vi "Open_abscisseSD.vi"(1 "wavelengths path":path) -> (0 "wavelengths":dbl[](array[numeric]) format="%.4f")   [LabVIEW 2015]
uses:
  <vilib>/Utility/file.llb/Read Delimited Spreadsheet (DBL).vi
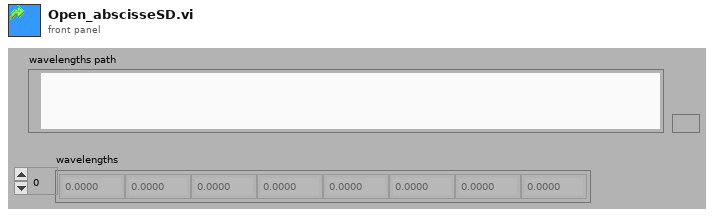
[diagram p1: front panel]
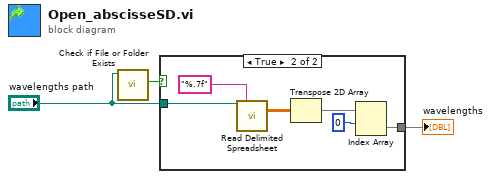
[diagram p0: block diagram]
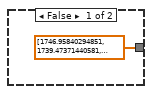
[diagram p2: hidden frame]
diagram:
  n1 = call <vilib>:"Check if File or Folder Exists.vi"("path"="wavelengths path") -> ("file or folder exists?"=w2:bool)  [unwired: 8 in, 2 out]
  n2 = case shown="True" w2 {
    tunnel: "wavelengths path" -> [_ w10]
    tunnel: [dbl[] [1746.95840294851, 1739.47371440581, 1731.99263543554, 1724.5156950524101, 1717.04336159476, 1709.5761853721801, 1702.1146510360302, 1694.65931938089, 1687.21070135242, 1679.76935602013, 1672.33583286395, 1664.91067290181, 1657.4944812369401, 1650.08777499183, 1642.69118936313, 1635.30526816863, 1627.93059787024, 1620.5678256451802, 1613.2174869458, 1605.8802162495501, 1598.55664914169, 1591.2473459440598, 1583.95293766588, 1576.67410341541, 1569.41139768648, 1562.16544706426, 1554.93690232794, 1547.72642715279, 1540.53459790541, 1533.3620467303099, 1526.2094059754, 1519.0773076058, 1511.96639712882, 1504.87731519191, 1497.81065537266, 1490.7670405046301, 1483.74708968683, 1476.7514175569002, 1469.7806335417001, 1462.8353410857799, 1455.91613685827, 1449.02362355376, 1442.1584350399, 1435.32109764276, 1428.5121745460801, 1421.73221797025, 1414.98176826326, 1408.2615312989599, 1401.57188671621, 1394.91332390898, 1388.2865399386899, 1381.69189429006, 1375.12987969607, 1368.60110805257, 1362.1058521608, 1355.64479016035, 1349.2181722474, 1342.8265206993399, 1336.47029749548, 1330.14974492859, 1323.8654016497699, 1317.61765329026, 1311.4067434369201, 1305.23303537283, 1299.0968750893198, 1292.99859208834, 1286.93855623105, 1280.91695705859, 1274.9340622176899, 1268.99011878883, 1263.0854499128502, 1257.2202233805301, 1251.39461273802, 1245.6087796279, 1239.86286216394, 1234.1571702132198, 1228.49182981838, 1222.8667403288, 1217.2823138311999, 1211.7384410115399, 1206.23526099378, 1200.77284844751, 1195.3512872829099, 1189.97039739273, 1184.63066565183, 1179.3316602586299, 1174.0734240220002, 1168.85619951437, 1163.6798326293401, 1158.54420056361, 1153.44927142328, 1148.3949947277902, 1143.3813012229598, 1138.40810270664, 1133.47529186764, 1128.58274213783, 1123.73030755832, 1118.9178226593901, 1114.1453578522999, 1109.41267699039, 1104.7194153073401, 1100.06545035942, 1095.4509959156, 1090.8752667265799, 1086.3386046025, 1081.8403792132801, 1077.38075829889, 1072.95905446028, 1068.5757295472001, 1064.22989459505, 1059.9215462309699, 1055.6507489056398, 1051.41685513876, 1047.2196667672001, 1043.05897437087, 1038.93469695662, 1034.84651523027, 1030.79405980805, 1026.7770747934799, 1022.79529322078, 1018.84843710765, 1014.93621751393, 1011.0584683138, 1007.2149741535, 1003.40527047478, 999.629026799409, 995.885902045937, 992.17596598108, 988.49879844413, 984.853757374839, 981.241054344726, 977.6601588227351, 974.110590515482, 970.592605892286, 967.1052106846611, 963.648839619437, 960.2226035956049, 956.826487302473, 953.460345239886, 950.123391218081, 946.8159012629151, 943.537424146781, 940.287407694674, 937.065621602715, 933.872182979098, 930.7066103284179, 927.568480301523, 924.4575441508091, 921.3735488679789, 918.3162372357681, 915.285347880829, 912.2806153275819, 909.3017700531, 906.348538542966, 903.420643348089, 900.517803142482, 897.639732781836, 894.786143363061, 891.956742284595, 889.151695015634, 886.370451849697, 883.6125789182599, 880.877770049898, 878.166234404625, 875.477603375355, 872.811181317668, 870.1671805836701, 867.5454303899451, 864.945008341113, 862.366773424345, 859.809471799701, 857.273487959592, 854.758299394799, 852.2638195761871, 849.789719421444, 847.335982951904, 844.901929890081, 842.488162930783, 840.093417182113, 837.718515604053, 835.362615919645, 833.025256625637, 830.707311695789, 828.407649933811, 826.1260369657721, 823.862809877985, 821.617722160325, 819.3901814280171, 817.180036573831, 814.9871818697229, 812.812007239723, 810.6537141958489, 808.512147956872, 806.3871529227789, 804.2785726895751, 802.186250064211, 800.1100270794481, 798.049745008728, 796.005244381085, 793.976454114127, 791.9630862877119, 789.964959427523, 787.981911065323, 786.0138311731309, 784.060630502893, 782.12207538586, 780.198000931301, 778.288241637713, 776.3926314076059, 774.511003562155, 772.643190855895, 770.789025491363, 768.948339133666, 767.121449826945, 765.307967824209, 763.507516369203, 761.719925215525, 759.945023646196, 758.1833910296, 756.4343900875849, 754.697623970222, 752.972920289276, 751.261192560027, 749.561354164361, 747.87311902268, 746.197142709487, 744.533015644908, 742.880029696423, 741.239027402037, 739.609387275517, 737.990423420732, 736.38361200569, 734.7872270711911, 733.201926757378, 731.6276420811399, 730.063551411954, 728.510886679627, 726.967845048158, 725.436176344851, 723.913978581447, 722.402723949191, 720.900885935728, 719.4097399027139, 717.9277761934089, 716.4564322952101, 714.9938562039661, 713.5420070365531, 712.098780852969, 710.6656679954409, 709.2415109958121, 707.8266171362831, 706.421219857516, 705.024166639125, 703.6371068683061, 702.258385108918, 700.888369872632, 699.527668337694, 698.175030143386, 696.8312120679619, 695.496163510531, 694.169015078566, 692.850439115762, 691.5404485401731, 690.238194392353, 688.94390353484, 687.658374393696, 686.3804175459129, 685.109988189973, 683.84778746451, 682.5935295926589, 681.3466345781219, 680.107057481696, 678.8753717724389, 677.6514112610839, 676.4346036036881, 675.224903742191, 674.0222665939291, 672.827515950317, 671.639819004719, 670.4590192709951, 669.28507156971, 668.117930701417, 666.957767455301, 665.804889055705, 664.658651647345, 663.5190099552269, 662.3859186887911, 661.259332542666, 660.1392061974129, 659.025494320265, 657.9185777458611, 656.818087211363, 655.723844942282, 654.635805560979, 653.553923680618, 652.4781539058861, 651.4084508336861, 650.34476905383, 649.287063149737, 648.235287699102, 647.1893972745651, 646.1493464444001, 645.1150897731491, 644.086581822294, 643.063777150895, 642.046630316235, 641.0350958744509, 640.029128381159, 639.028682392086, 638.0337124636501, 637.0441731536, 636.060019021599, 635.081204629804, 634.107684543462, 633.1394133314781, 632.176345566988, 631.2184358279051, 630.265638697489, 629.317908764871, 628.375200625596, 627.437468882152, 626.504668144487, 625.576753030516, 624.653678166628, 623.735398188169, 622.821867739936, 621.913041476642, 621.0089253567401, 620.109953829607, 619.2155803341301, 618.325759554615, 617.440446187314, 616.559594940844, 615.68316053661, 614.8110977092091, 613.943361206831, 613.080378184452, 612.2219946300979, 611.367831427453, 610.517843366502, 609.67198525252, 608.83021190643, 607.99247816513, 607.1596936044419, 606.33093309446, 605.506106395553, 604.685168394393, 603.868073995068, 603.05511142711, 602.246732258074, 601.442091036539, 600.6411427211999, 599.843842289426, 599.050453455946, 598.261610552242, 597.476310031922, 596.694506931211, 595.916156306054, 595.142093000695, 594.371942537607, 593.6051392171811, 592.8416381578529, 592.0819061727381, 591.326408617177, 590.574108124154, 589.82495987703, 589.079419713967, 588.338078537831, 587.5997845495849, 586.864492999568, 586.1330052374029, 585.405324564155, 584.6805414170831, 583.9586111151431, 583.2410364251999, 582.526521056125, 581.8147537706529, 581.106377109973, 580.40188911896, 579.700044555559, 579.000804083577, 578.3061033013261, 577.613941398089, 576.924273860396, 576.238621805796, 575.5559027380571, 574.875573645619, 574.198903353956, 573.525387538455, 572.854157418386, 572.186407197363, 571.521855295781, 570.859484920937, 570.200593127219, 569.544766049075, 568.89101644063, 568.24092148275, 567.593580387639, 566.9482128169841, 566.306853158223, 565.6677594573711, 565.030744389789, 564.397849608573, 563.766764965671, 563.1383930010489, 562.5133728535751, 561.890059184882, 561.270268935877, 560.652885480491, 560.037363089153, 559.425835098158, 558.8158506451961, 558.208818010672, 557.604554961745, 557.001744243597, 556.40312797365, 555.805892569102, 555.2114798040269, 554.619757339678, 554.0295206295671, 553.443236604538, 552.858171035084, 552.276240638747, 551.696479889713, 551.118679771488, 550.544149465713, 549.970675460912, 549.401090190914, 548.832713227076, 548.267212547523, 547.703858369913, 547.1424270722009, 546.584021469991, 546.0266443561001, 545.473113162201, 544.9203584328391, 544.371044135748, 543.823030776167, 543.2777251340771, 542.734379095834, 542.193066954772, 541.6543142319989, 541.116980449427, 540.582747078486, 540.04937652346, 539.519588582563, 538.9902391902291, 538.464749744689, 537.93971315779, 537.418141618218, 536.89734402556, 536.37967530906, 535.86304293919, 535.349261975299, 534.836721095929, 534.326812826771, 533.818289744137, 533.312239124593, 532.8076601827761, 532.305452180648, 531.804743760851, 531.306363357019, 530.809451876789, 530.3148840653839, 529.8216959777941, 529.330925766354, 528.841387559125, 528.3543999687649, 527.8684381633481, 527.385218228913, 526.9027593795071, 526.4232921497451, 525.944262842272, 525.468533379988, 524.992860231003, 524.520853613227, 524.0488469954499, 523.58016458692, 523.1118659050629, 522.6463780813681, 522.181772441391, 521.719405918609, 521.2584784411761, 520.79915996126, 520.341895781911, 519.8855521113021, 519.4319363806011, 518.9784943087769, 518.528512192482, 518.078530076188, 517.631535209674, 517.185171888899, 516.7409174597481, 516.298158131117, 515.85657100424, 515.417400880057, 514.978407937087, 514.542812245489, 514.107216553891, 513.674304368112, 513.242268353238, 512.811789417832, 512.3832983399769, 511.95517959197304, 511.53021872775594, 511.105257863537, 510.682941755925, 510.26149639844397, 509.84137968758904, 509.42343514659206, 509.005490605594, 508.590986409599] ("x*y") w5] -> w1
    frame False {
    }
    frame True {
      n3 = call-poly <vilib>:"Read Delimited Spreadsheet.vi"("file path (dialog if empty)"=w10, "format (%.3f)"="%.7f") -> ("all rows"=w6:dbl[][])  [unwired: 8 in, 5 out]
      n4 = Transpose 2D Array(2D array=w6) -> (transposed array=w7:dbl[][])
      n5 = Index Array(array=w7, index (row)=0) -> (element=w5:dbl[])  [unwired: 1 in]
    }
  }
  "wavelengths" <- w1
